vi "Open and Configure Device Core.vi"(0 "USRP RIO Device":T3, 1 "reference frequency source":string(combo)="Internal", 3 "which bitfile":string(combo)="Time", 4 "wait for gps lock?":bool, 5 "error in":errorcluster, 6 "Rx?":bool, 7 "rx config":T5={"channel configuration"=[], "transfer mode"=enum."Finite", "sample rate"=10000000.0, "number of samples"=8192, "start trigger"=enum."Immediate"} {"channel configuration"."channel configuration"."frequency" format="%#.3pHz"; "channel configuration"."channel configuration"."lo frequency" format="%#.3pHz"; "channel configuration"."channel configuration"."level" format="%#_gdBm"; "sample rate" format="%#.3pS/s"}, 11 "tx config":T6={"channel configuration"=[], "transfer mode"=enum."Finite", "sample rate"=10000000.0, "number of samples"=8192, "start trigger"=enum."Immediate", "tone frequency"=100000.0} {"channel configuration"."channel configuration"."frequency" format="%#.3pHz"; "channel configuration"."channel configuration"."lo frequency" format="%#.3pHz"; "channel configuration"."channel configuration"."level" format="%#_gdBm"; "tone frequency" format="%#.3pHz"; "sample rate" format="%#.3pS/s"}, 13 "lo config":T2) -> (10 "rx channels":T8={"rx config"={"channel configuration"=[], "transfer mode"=enum."Finite", "sample rate"=10000000.0, "number of samples"=8192, "start trigger"=enum."Immediate"}, "reference frequency source"="Internal", "rx.data sink"=enum."Host", "rx.enabled channels"=[], "vertical range"=[], "rx.coerced configurations"={"coerced frequencies"=[], "coerced lo frequencies"=[], "coerced levels"=[], "coerced sample rates"=[]}} {"rx.coerced configurations"."coerced sample rates" format="%#.3pS/s"; "rx.coerced configurations"."coerced levels" format="%#.3gdBm"; "rx.coerced configurations"."coerced lo frequencies" format="%#.3pHz"; "rx.coerced configurations"."coerced frequencies" format="%#.3pHz"; "rx config"."channel configuration"."channel configuration"."frequency" format="%#.3pHz"; "rx config"."channel configuration"."channel configuration"."lo frequency" format="%#.3pHz"; "rx config"."channel configuration"."channel configuration"."level" format="%#_gdBm"; "rx config"."sample rate" format="%#.3pS/s"; "vertical range" format="%#.3pVpp"}, 12 "tx channels":T7={"tx config"={"channel configuration"=[], "transfer mode"=enum."Finite", "sample rate"=10000000.0, "number of samples"=8192, "start trigger"=enum."Immediate", "tone frequency"=100000.0}, "reference frequency source"="Internal", "tx.data source"=enum."Host", "tx.enabled channels"=[], "I"=[], "Q"=[], "tx.coerced configurations"={"coerced frequencies"=[], "coerced lo frequencies"=[], "coerced levels"=[], "coerced sample rates"=[]}} {"tx.coerced configurations"."coerced sample rates" format="%#.3pS/s"; "tx.coerced configurations"."coerced levels" format="%#.3gdBm"; "tx.coerced configurations"."coerced lo frequencies" format="%#.3pHz"; "tx.coerced configurations"."coerced frequencies" format="%#.3pHz"; "tx config"."channel configuration"."channel configuration"."frequency" format="%#.3pHz"; "tx config"."channel configuration"."channel configuration"."lo frequency" format="%#.3pHz"; "tx config"."channel configuration"."channel configuration"."level" format="%#_gdBm"; "tx config"."tone frequency" format="%#.3pHz"; "tx config"."sample rate" format="%#.3pS/s"}, 14 "niUsrpRio Session (out)":T10 {"Daughterboard Clock Rate" format="%#.3pHz"; "FPGA Data Clock Rate" format="%#.3pHz"; "Data Clock Rate" format="%#.3pHz"; "Characterization Data"."Frequencies [Hz]" format="%#_6p"; "EEPROM Characterization Header"."Pointer to Device Data Header" format="%x"; "EEPROM Characterization Header"."Checksum" format="%x"; "Device Data Header"."Pointer to Characterization Data" format="%x"; "Device Data Header"."Checksum" format="%x"; "EEPROM Header"."Pointer to User Header" format="%x"; "EEPROM Header"."Pointer to Factory Header" format="%x"; "EEPROM Header"."Product Code" format="%x"; "EEPROM Header"."Checksum" format="%x"}, 15 "rx.coerced configurations":T9 {"coerced sample rates" format="%#.3pS/s"; "coerced levels" format="%#.3gdBm"; "coerced lo frequencies" format="%#.3pHz"; "coerced frequencies" format="%#.3pHz"}, 16 "tx.output waveform":waveform(dbl)[](graph), 17 "tx.coerced configurations":T9 {"coerced sample rates" format="%#.3pS/s"; "coerced levels" format="%#.3gdBm"; "coerced lo frequencies" format="%#.3pHz"; "coerced frequencies" format="%#.3pHz"}, 18 "Ports debug":T1(array[cluster]), 19 "error out":errorcluster)   [LabVIEW 2016]
uses:
  <instrlib>/niUsrpRio/Config/v1/Host/Public/niUsrpRio Session.ctl
  <instrlib>/_niInstr/Register Bus/v0/Host/Public/Register Bus Session.ctl
  <instrlib>/_niInstr/Register Bus/v0/Host/Private/Session Data.ctl
  <instrlib>/niUsrpRio/Config/v1/Host/Private/DB Queue Reference.ctl
  <instrlib>/niUsrpRio/Config/v1/Host/Private/Daughterboard Data.ctl
  <instrlib>/niUsrpRio/Config/v1/Host/Private/ATR state data.ctl
  <instrlib>/niUsrpRio/Config/v1/Host/Private/Antenna Configuration.ctl
  <instrlib>/niUsrpRio/Config/v1/Host/Private/CPLD Power Mode.ctl
  <instrlib>/niUsrpRio/Config/v1/Host/Public/EEPROM Header.ctl
  <instrlib>/niUsrpRio/Config/v1/Host/Public/EEPROM Device Data Header.ctl
  <instrlib>/niUsrpRio/Config/v1/Host/Public/EEPROM Characterization Header.ctl
  <instrlib>/niUsrpRio/Config/v1/Host/Public/Characterization Data.ctl
  <instrlib>/niUsrpRio/Config/v1/Host/Public/IQ Imbalance.ctl
  Rx Channels.ctl
  Start Trigger.ctl
  Tx Channels.ctl
  <vilib>/userdefined/Silver/nirio_resource_slv.ctl
  <instrlib>/_niInstr/Register Bus/v0/Host/niInstr Register Bus v0 Host.lvlib
  <instrlib>/niUsrpRio/Config/v1/Host/niUsrpRio Config v1 Host.lvlib
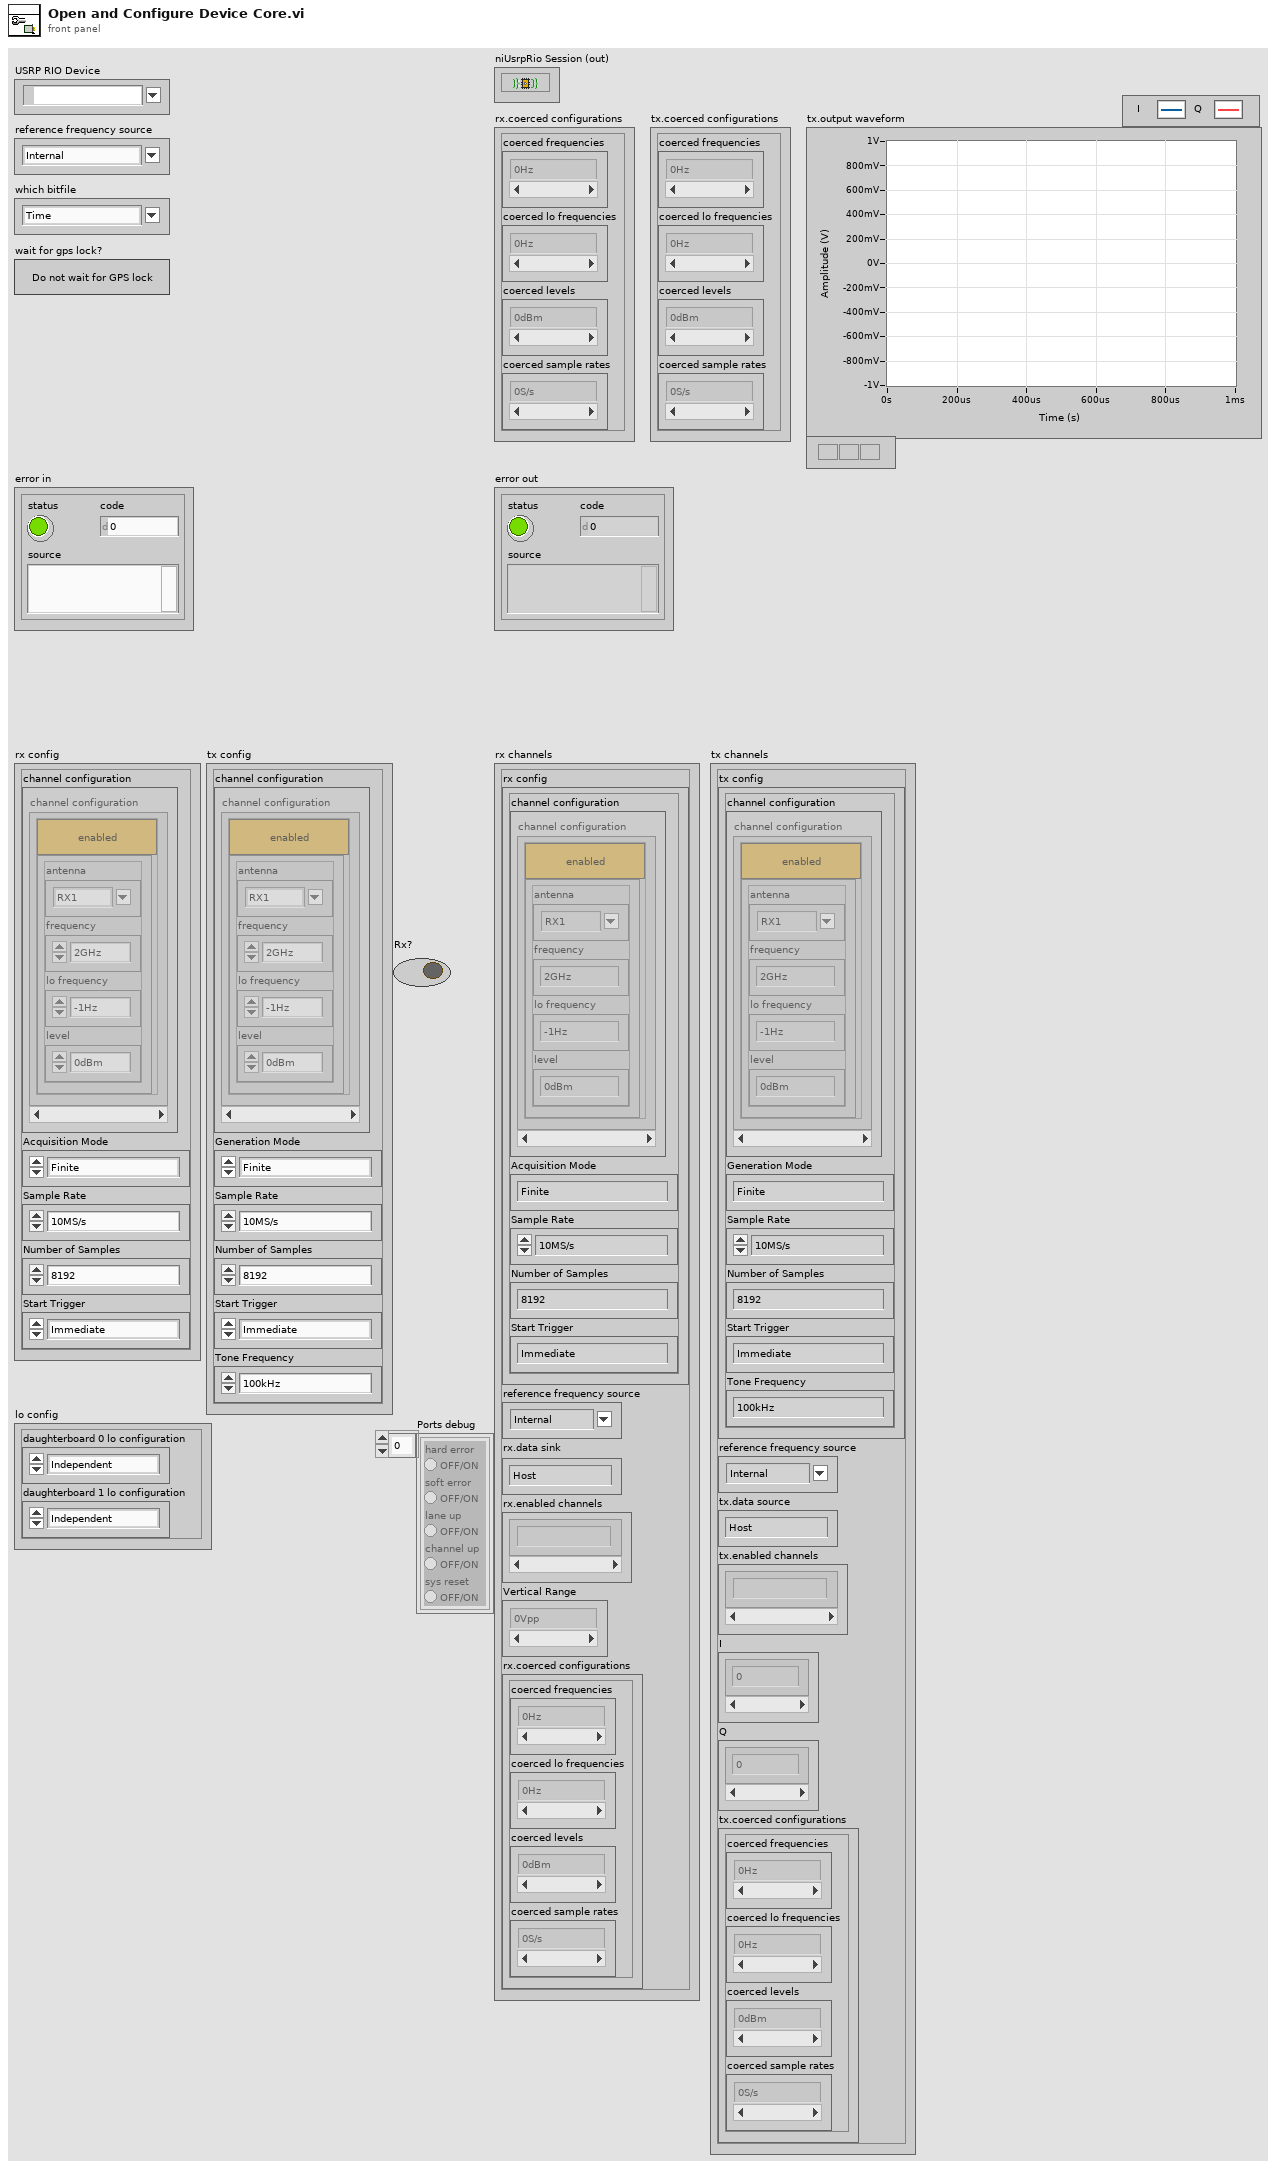
[diagram p1: front panel]
types:
  T1 = cluster{"hard error":bool, "soft error":bool, "lane up":bool, "channel up":bool, "sys reset":bool}[]
  T2 = cluster{"daughterboard 0 lo configuration":enum16{"Independent", "Import", "Shared and Export"}, "daughterboard 1 lo configuration":enum16{"Independent", "Import", "Shared and Export"}}
  T3 = typedef "nirio_resource_slv.ctl" = tag
  T4 = typedef "Start Trigger.ctl" = enum8{"Software", "Digital Edge", "Rx Start Trigger", "Tx Start Trigger", "Immediate", "Future Time Event"}
  T5 = cluster{"channel configuration":cluster{"channel enable":bool, "channel configuration":cluster{"antenna":string, "frequency":dbl, "lo frequency":dbl, "level":dbl}}[], "transfer mode":enum16{"Finite", "Continuous"}, "sample rate":dbl, "number of samples":u32, "start trigger":T4}
  T6 = cluster{"channel configuration":cluster{"channel enable":bool, "channel configuration":cluster{"antenna":string, "frequency":dbl, "lo frequency":dbl, "level":dbl}}[], "transfer mode":enum16{"Finite", "Continuous"}, "sample rate":dbl, "number of samples":u32, "start trigger":T4, "tone frequency":dbl}
  T7 = typedef "Tx Channels.ctl" = cluster{"tx config":cluster{"channel configuration":cluster{"channel enable":bool, "channel configuration":cluster{"antenna":string, "frequency":dbl, "lo frequency":dbl, "level":dbl}}[], "transfer mode":enum16{"Finite", "Continuous"}, "sample rate":dbl, "number of samples":u32, "start trigger":T4, "tone frequency":dbl}, "reference frequency source":string, "tx.data source":enum16{"SFP Port 0", "SFP Port 1", "Host"}, "tx.enabled channels":string[], "I":i16[], "Q":i16[], "tx.coerced configurations":cluster{"coerced frequencies":dbl[], "coerced lo frequencies":dbl[], "coerced levels":dbl[], "coerced sample rates":dbl[]}}
  T8 = typedef "Rx Channels.ctl" = cluster{"rx config":cluster{"channel configuration":cluster{"channel enable":bool, "channel configuration":cluster{"antenna":string, "frequency":dbl, "lo frequency":dbl, "level":dbl}}[], "transfer mode":enum16{"Finite", "Continuous"}, "sample rate":dbl, "number of samples":u32, "start trigger":T4}, "reference frequency source":string, "rx.data sink":enum16{"SFP Port 0", "SFP Port 1", "Host"}, "rx.enabled channels":string[], "vertical range":dbl[], "rx.coerced configurations":cluster{"coerced frequencies":dbl[], "coerced lo frequencies":dbl[], "coerced levels":dbl[], "coerced sample rates":dbl[]}}
  T9 = cluster{"coerced frequencies":dbl[], "coerced lo frequencies":dbl[], "coerced levels":dbl[], "coerced sample rates":dbl[]}
  T10 = typedef "niUsrpRio Config v1 Host.lvlib/niUsrpRio Session.ctl" = cluster{"FPGA Interface":refnum<k20>, "RIO Interface Number":u32, "Data Clock Rate":u32, "FPGA Data Clock Rate":u32, "Global Settings Register Bus":T11, "Radio 0 Settings Register Bus":T11, "Radio 1 Settings Register Bus":T11, "Radio Settings Bus Semaphore":T12, "DB Queues":T13[], "Characterization Data Valid?":bool, "EEPROM Header":T14, "Device Data Header":T15, "EEPROM Characterization Header":T16, "Characterization Data":T17[], "FPGA Current Version":u32, "FPGA Oldest Compatible Version":u32, "Fixed Logic Current Version":u32, "Fixed Logic Oldest Compatible Version":u32, "FPGA Radio Settings Bus Current Version":u32, "FPGA Radio Settings Bus Oldest Compatible Version":u32, "FPGA Board Config Current Version":u32, "FPGA Board Config Oldest Compatible Version":u32, "Daughterboard Clock Rate":u32, "daughterboard configuration session handles":u64[]}
  T11 = typedef "niInstr Register Bus v0 Host.lvlib/Register Bus Session.ctl" = refnum<queue>
  T12 = typedef "Semaphore RefNum" = refnum<k1>
  T13 = typedef "niUsrpRio Config v1 Host.lvlib/DB Queue Reference.ctl" = refnum<queue>
  T14 = typedef "niUsrpRio Config v1 Host.lvlib/EEPROM Header.ctl" = cluster{"Checksum":u32, "Product Code":u16, "Hardware Current Version":u16, "Hardware Oldest Compatible Version":u16, "EEPROM Map Current Version":u16, "EEPROM Map Oldest Compatible Version":u16, "User Password":string, "Pointer to Factory Header":u32, "Pointer to User Header":u32, "Recommended Interval":u16, "Number of Reserved Bytes":i32, "Number of Daughterboards":u8, "Daughterboard IDs":u16[], "Daughterboard Serial Numbers":string[]}
  T15 = typedef "niUsrpRio Config v1 Host.lvlib/EEPROM Device Data Header.ctl" = cluster{"Checksum":u32, "Number of Channels":u8, "Number of Gain Settings":u16[], "Pointer to Characterization Data":u32[], "Number of Reserved Bytes":i32, "Number of Frequencies":u16[]}
  T16 = typedef "niUsrpRio Config v1 Host.lvlib/EEPROM Characterization Header.ctl" = cluster{"Checksum":u32, "Date":timestamp, "Temperature":sgl, "Misc. Info":string, "Pointer to Device Data Header":u32, "Number of Reserved Bytes":i32}
  T17 = typedef "niUsrpRio Config v1 Host.lvlib/Characterization Data.ctl" = cluster{"Gains[dB]":dbl[], "Frequencies [Hz]":dbl[], "IQ Imbalance Table":T18[], "Measured Gains[dB]":dbl[][]}
  T18 = typedef "niUsrpRio Config v1 Host.lvlib/IQ Imbalance.ctl" = cluster{"Gain Imbalance [linear]":dbl, "Phase Imbalance [radians]":dbl, "Offset":cdb}
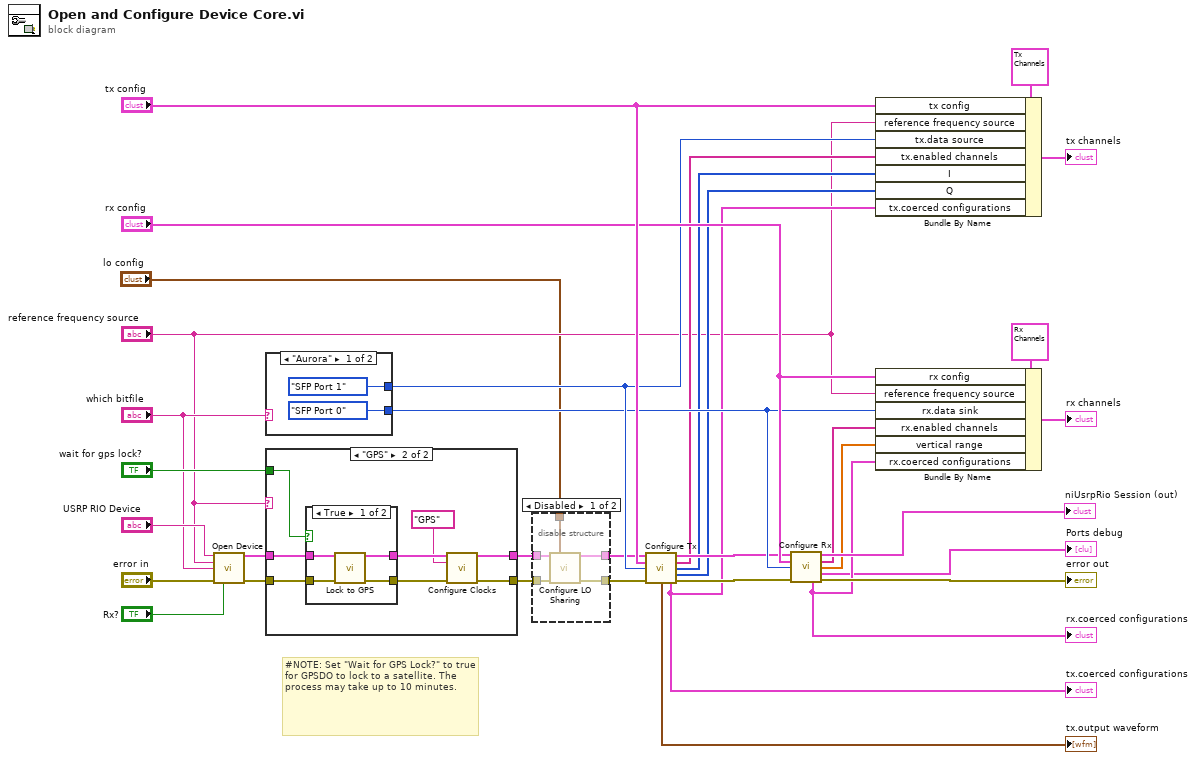
[diagram p0: block diagram]
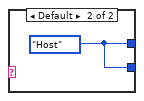
[diagram p3: hidden frame]
diagram:
  # "#NOTE: Set \"Wait for GPS Lock?\" to true for GPSDO to lock to a satellite. The process may take up to 10 minutes."
  n1 = call "Open Device.vi"("USRP RIO device"="USRP RIO Device", "Rx?"="Rx?", "Reference Frequency Source"="reference frequency source", "which bitfile"="which bitfile", "error in"="error in") -> ("niUsrpRio Session (out)"=w13:T10, "error out"=w12:errorcluster)  [unwired: 9 in]
  n2 = case shown="\"Aurora\"" "which bitfile" {
    tunnel: [enum16{"SFP Port 0", "SFP Port 1", "Host"}."SFP Port 1" ("data stream config") w37] -> w30
    tunnel: [enum16{"SFP Port 0", "SFP Port 1", "Host"}."SFP Port 0" ("data stream config") w37] -> w29
    frame "Aurora" {
    }
    frame Default {
      w37 = enum16{"SFP Port 0", "SFP Port 1", "Host"}."Host" ("data stream config")
    }
  }
  n3 = case shown="\"GPS\"" "reference frequency source" {
    tunnel: w13 -> [w39 w47]
    tunnel: [w39 w42] -> w6
    tunnel: [w38 w44] -> w5
    tunnel: w12 -> [w38 w46]
    tunnel: "wait for gps lock?" -> [_ w40]
    frame Default {
    }
    frame "GPS" {
      n4 = case shown="True" w40 {
        tunnel: w47 -> [w49 w53]
        tunnel: [w51 w53] -> w43
        tunnel: [w50 w52] -> w45
        tunnel: w46 -> [w48 w52]
        frame True {
          n5 = call "Lock to GPS.vi"("niUsrpRio Session"=w49, "error in"=w48) -> ("niUsrpRio Session (out)"=w51:T10, "error out"=w50:errorcluster)  [unwired: 12 in]
        }
        frame False {
        }
      }
      n6 = call "Configure Clocks.vi"("niUsrpRio Session"=w43, "Reference Frequency Source"="GPS", "error in"=w45) -> ("niUsrpRio Session (out)"=w42:T10, "error out"=w44:errorcluster)  [unwired: 11 in]
    }
  }
  n7 = disable-structure shown="Disabled" {
    disable-tunnel: [w58 w60] -> w7
    disable-tunnel: w6 -> [w57 w60]
    disable-tunnel: w5 -> [w56 w59]
    disable-tunnel: [w55 w59] -> w4
    disable-tunnel: "lo config" -> [w54 _]
    frame Disabled {
      n8 = call "Configure LO Sharing.vi"("niUsrpRio Session in"=w57, "lo config"=w54, "error in"=w56) -> ("niUsrpRio Session out"=w58:T10, "error out"=w55:errorcluster)  [unwired: 11 in]
    }
    frame Enabled {
    }
  }
  n9 = call "Configure Tx.vi"("niUsrpRio Session"=w7, "tx config"="tx config", "tx.data source"=w30, "error in"=w4) -> ("niUsrpRio Session (out)"=w21:T10, "tx.enabled channels"=w17:string[], "I"=w18:i16[], "Q"=w19:i16[], "tx.output waveform"=→"tx.output waveform":waveform(dbl)[], "tx.coerced configurations"=w20:T9, "error out"=w22:errorcluster)  [unwired: 5 in]
  "tx.coerced configurations" <- w20
  n10 = call "Configure Rx.vi"("niUsrpRio Session"=w21, "rx config"="rx config", "rx.data sink"=w29, "error in"=w22) -> ("niUsrpRio Session (out)"=→"niUsrpRio Session (out)":T10, "rx.enabled channels"=w26:string[], "vertical range"=w25:dbl[], "Ports debug"=→"Ports debug":T1, "rx.coerced configurations"=w23:T9, "error out"=→"error out":errorcluster)  [unwired: 6 in]
  "rx.coerced configurations" <- w23
  n11 = Bundle By Name(cluster=T7 {"tx config"={"channel configuration"=[], "transfer mode"=enum."Finite", "sample rate"=10000000.0, "number of samples"=8192, "start trigger"=enum."Immediate", "tone frequency"=100000.0}, "reference frequency source"="Internal", "tx.data source"=enum."Host", "tx.enabled channels"=[], "I"=[], "Q"=[], "tx.coerced configurations"={"coerced frequencies"=[], "coerced lo frequencies"=[], "coerced levels"=[], "coerced sample rates"=[]}} ("tx channels"), "tx config"="tx config", "reference frequency source"="reference frequency source", "tx.data source"=w30, "tx.enabled channels"=w17, "I"=w18, "Q"=w19, "tx.coerced configurations"=w20) -> (→"tx channels":T7)
  n12 = Bundle By Name(cluster=T8 {"rx config"={"channel configuration"=[], "transfer mode"=enum."Finite", "sample rate"=10000000.0, "number of samples"=8192, "start trigger"=enum."Immediate"}, "reference frequency source"="Internal", "rx.data sink"=enum."Host", "rx.enabled channels"=[], "vertical range"=[], "rx.coerced configurations"={"coerced frequencies"=[], "coerced lo frequencies"=[], "coerced levels"=[], "coerced sample rates"=[]}} ("rx channels"), "rx config"="rx config", "reference frequency source"="reference frequency source", "rx.data sink"=w29, "rx.enabled channels"=w26, "vertical range"=w25, "rx.coerced configurations"=w23) -> (→"rx channels":T8)
